vi "D3DM.vi"() -> ()   [LabVIEW 2013]
uses:
  <vilib>/Native 3D Graph/xcontrol/3DPC_SurfacePlot.xctl
  <vilib>/Platform/NI_3dgraph.lvlib
panel:
  out "String":string
  in  "Tab Control":T1(tab)
  in  "mode":enum16{"Manual", "Quad", "Vertical", "Half"}(ring)
  in  "Byte to Read(TCP)":i32=512
  in  "Port":u16=8899
  in  "Log File Path":path=path "E:/Dropbox/StaredProject/Distributed3D/D3DM/raw_log.txt"
  in  "Simulation":bool
  out "Init Status":bool
  in  "User Param 2":i16=3000
  in  "User Param 1":i16=1024
  in  "holder_length":dbl=87.37
  in  "magOffset 1":i16
  in  "magOffset 2":i16=-1725
  in  "Servo":i16[](array[numeric])=[1000, 2000, 600, 2190, 1475]
  in  "ArcStepThreshold":dbl=800000.0
  in  "Least Dis":dbl=240.0
  out "InRange":bool
  out "Points Number":i32
  in  "3D Curve - Lorenz Attractor":refnum<k7>(container)
  in  "Arm Angle Set":i32(slide)=90 min=0 max=180 scale=0.0..180.0
  out "Title":string="      Distributed 3D Measurement Control Panel"
  in  "Initialize":bool
  in  "Base Rotation Speed Set":i32(slide)=1475 min=1000 max=2000 step=1 scale=1000.0..2000.0
  in  "Command":string
  out "Read Buffer":string
  out "help":string="1.Set the target Port number;\n2.Press \"Ready\" button to start acquiring data;\n3.Use arrow keys to control movement;\n4.Use the speed pointer slide to control speed;\n5.Use the Arm Angle slide to control arm;\n6.Press \"ESC\" to stop the car, 3D plot should be     finished automatically.\n\n//quad parameters\nint leftLimit = 1024;\nint rightLimit = 3072;\n//vertical parameters\nint vertical_delay_time = 100;\nint vertical_spd = BASE_STOP + 150;\n//half parameters\nint half_spd = BASE_STOP + 150;\nint half_angle_step = 1;"
  out "3D Graph":refnum<class "Base Datatype.lvclass">[](xcontrol)
  in  "Stop Button":bool
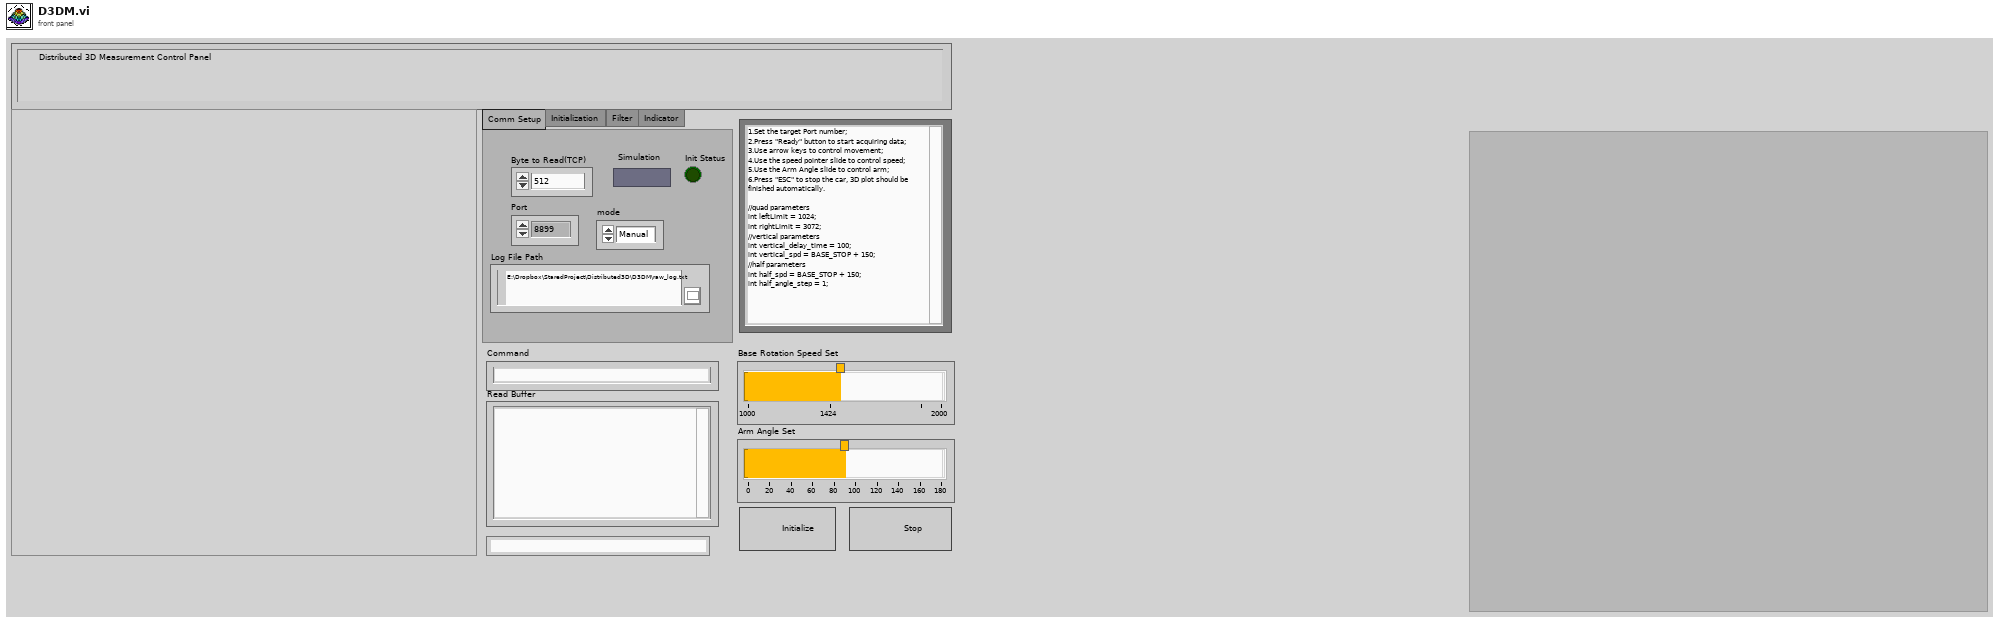
[diagram p1: front panel]
types:
  T1 = enum32{"Comm Setup", "Initialization", "Filter", "Indicator"}
  T2 = enum16{"open", "replace", "create", "open or create", "replace or create", "replace or create with confirmation"}
  T3 = enum16{"Standard", "Buffered", "CRLF", "Immediate"}
  T4 = typedef "eventvkey.ctl" = enum16{"ASCII", "Enter", "Return", "Shift", "Ctrl", "Alt", "Cmd", "Opt", "Caps", "NumLock", "Clear", "Break", "Up", "Down", "Left", "Right", "Insert", "Delete", "Home", "End", "PageUp", "PageDown", "Escape", "Help", "Pause", "ScrollLock", "F1", "F2", "F3", "F4", "F5", "F6", "F7", "F8", "F9", "F10", "F11", "F12", "F13", "F14", "F15", "F16", "F17", "F18", "F19", "F20", "F21", "F22", "F23", "F24", "Play", "VolumeUp", "VolumeDown", "Mute", "Two Byte Char"}
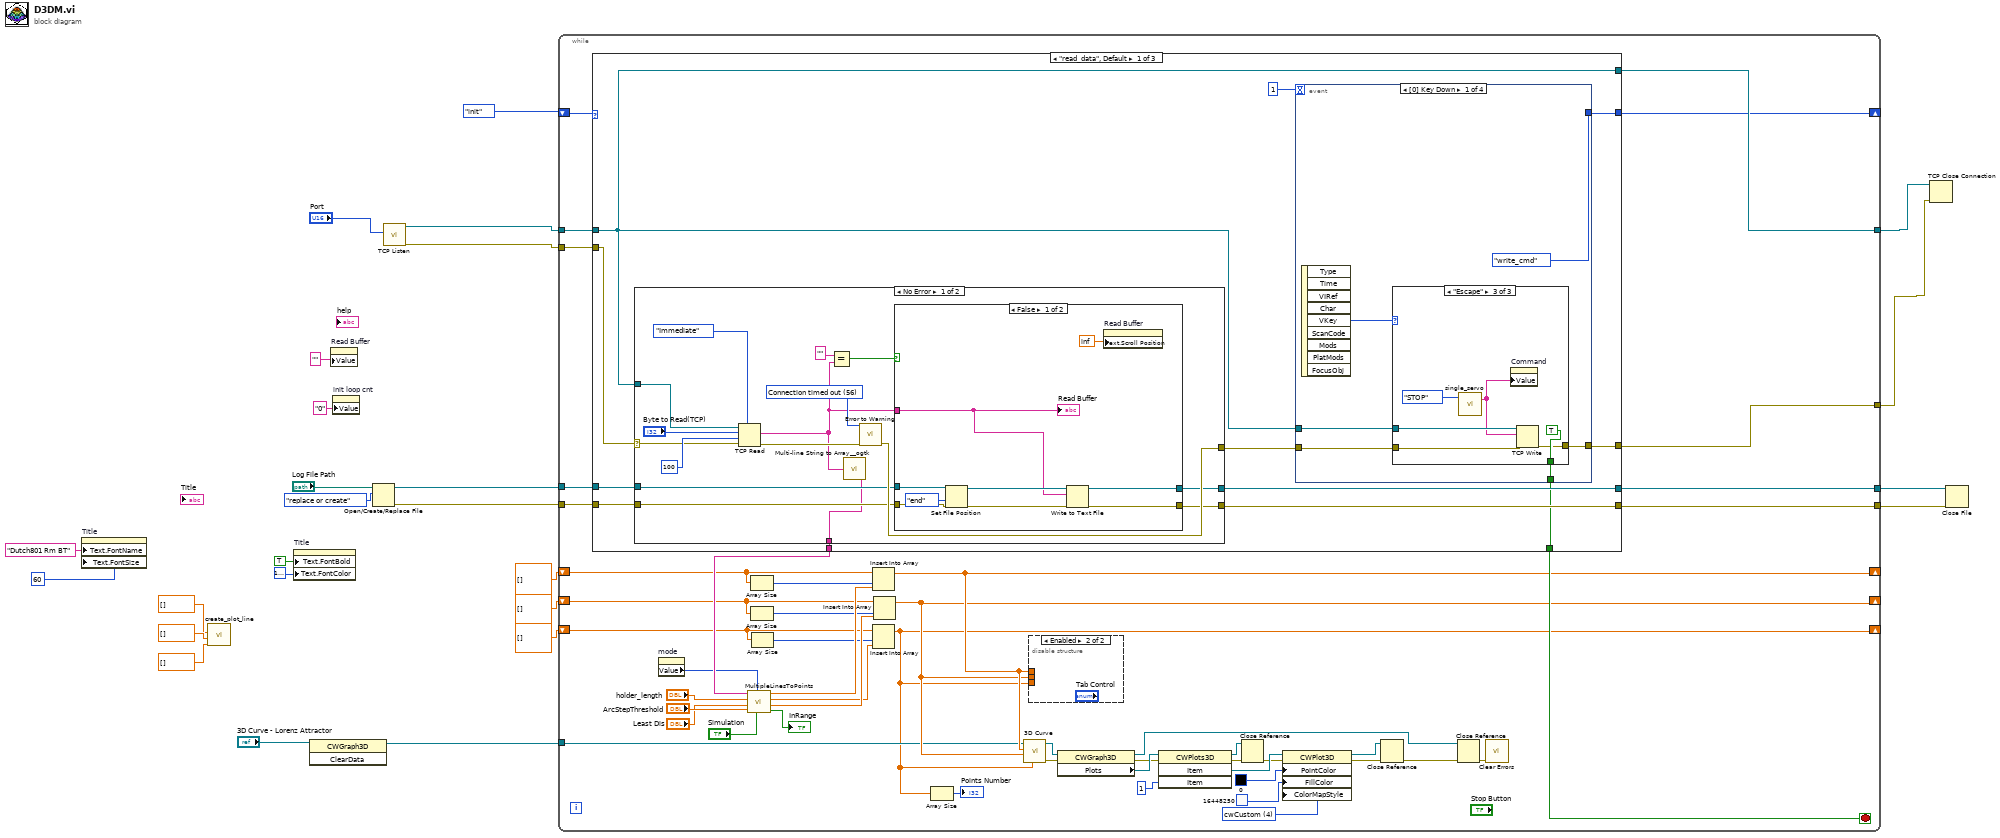
[diagram p0: block diagram]
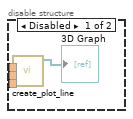
[diagram p2: hidden frame]
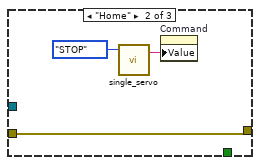
[diagram p4: hidden frame]
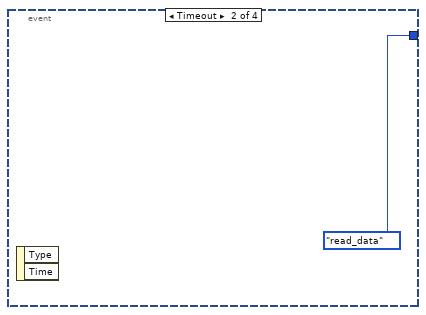
[diagram p5: hidden frame]
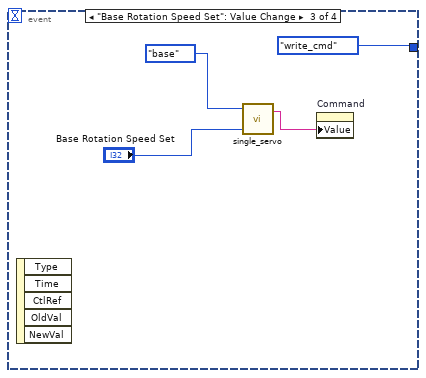
[diagram p6: hidden frame]
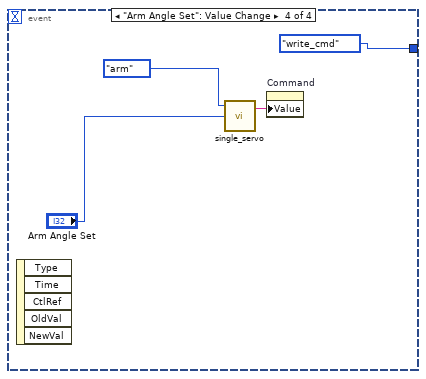
[diagram p7: hidden frame]
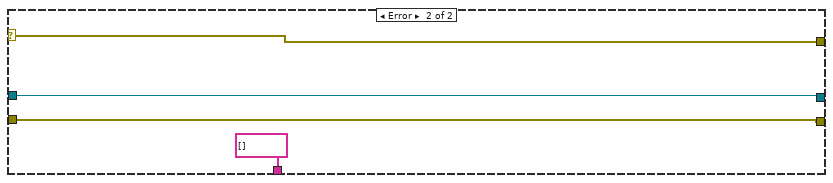
[diagram p9: hidden frame]
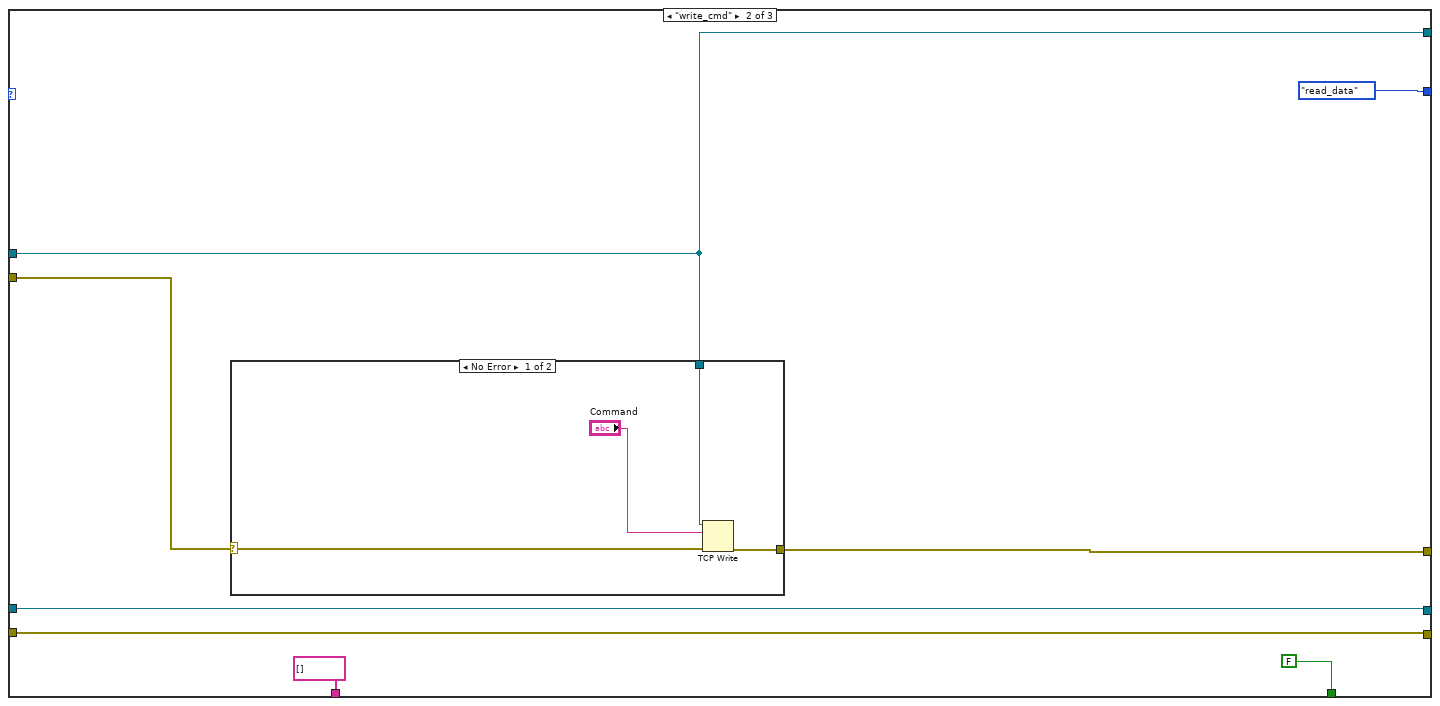
[diagram p10: hidden frame]
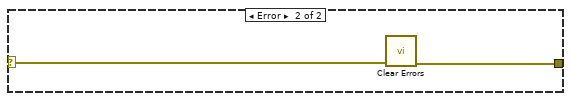
[diagram p11: hidden frame]
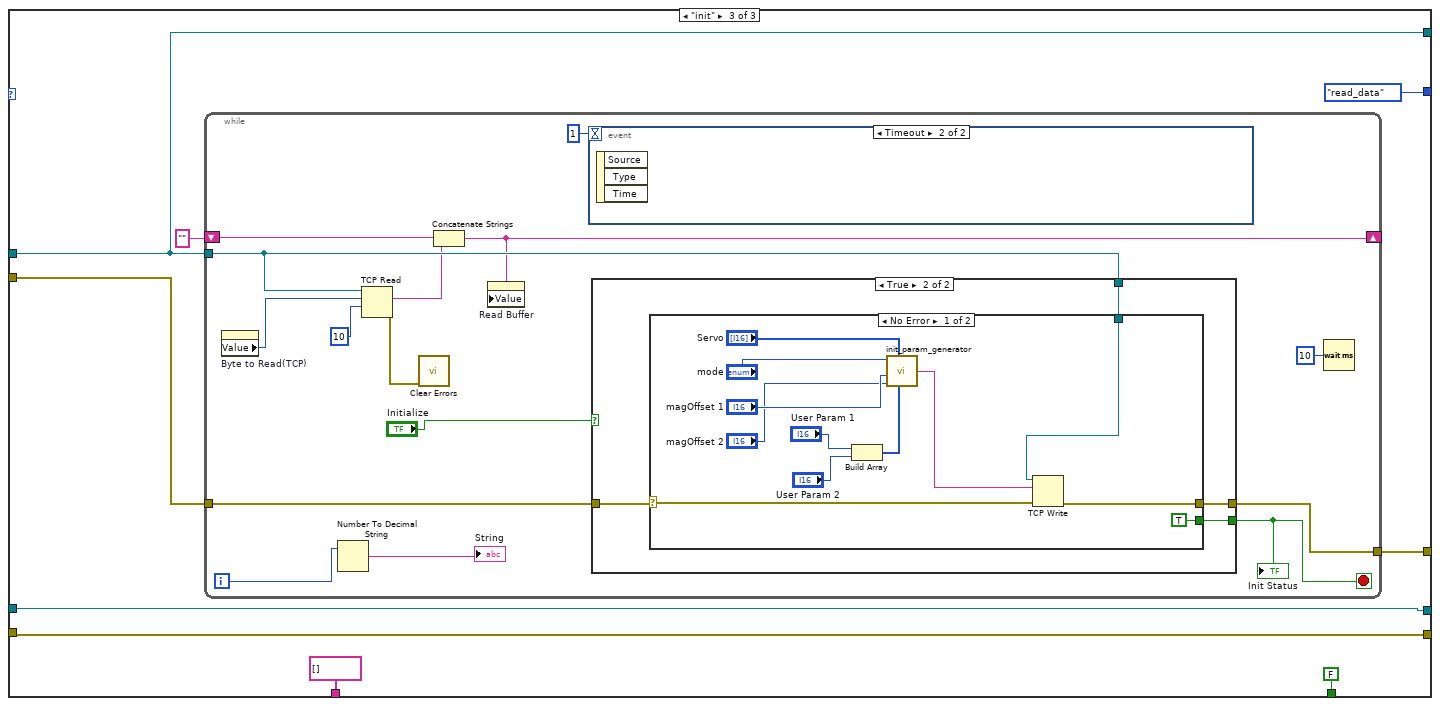
[diagram p12: hidden frame]
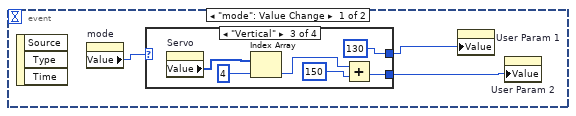
[diagram p13: hidden frame]
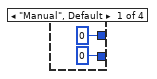
[diagram p14: hidden frame]
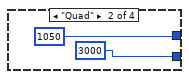
[diagram p15: hidden frame]
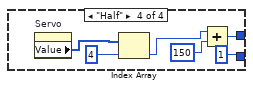
[diagram p16: hidden frame]
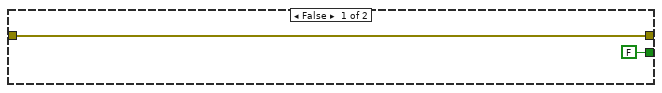
[diagram p17: hidden frame]
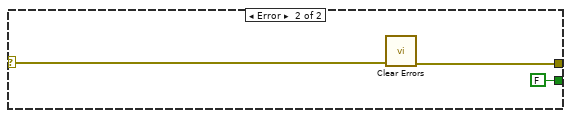
[diagram p18: hidden frame]
diagram:
  n1 = property on="Title" class="Str"("Text.FontName"="Dutch801 Rm BT" ("Text.Font:Name"), "Text.FontSize"=u32 60 ("Text.Font:Size")) -> ()  [unwired: 2 in, 2 out]
  n2 = call <vilib>:"create_plot_line.vi"("z vector"=dbl[] [], "y vector"=dbl[] [], "x vector"=dbl[] []) -> ()  [unwired: 8 in, 1 out]
  n3 = property on="Title" class="Str"("Text.FontBold"=TRUE ("Text.Font:Bold"), "Text.FontColor"=u32 16777222) -> ()  [unwired: 2 in, 2 out]
  n4 = invoke class="CWGraph3D" method="ClearData"(reference="3D Curve - Lorenz Attractor") -> (reference out=w6:refnum<k7>)  [unwired: 2 in, 2 out]
  n5 = property on="Read Buffer" class="Str"("Value"="") -> ()  [unwired: 2 in, 2 out]
  n6 = property on="init loop cnt" class="Str"("Value"="0" ("String")) -> ()  [unwired: 2 in, 2 out]
  n7 = Open/Create/Replace File(file path (use dialog)="Log File Path", operation (0:open)=T2."replace or create") -> (refnum out=w19:refnum<file>, error out=w18:errorcluster)  [unwired: 4 in, 1 out]
  n8 = call <vilib>:"TCP Listen.vi"("port"="Port") -> ("error out"=w24:errorcluster, "connection ID"=w25:refnum<k5>)  [unwired: 6 in, 3 out]
  n9 = while {
    shift-right: [w65] -> _
    shift-left: enum16{"read_data", "write_cmd", "init"}."init" ("RWstate") -> [w75]
    tunnel: w24 -> [w74]
    tunnel: w25 -> [w73]
    tunnel: w19 -> [w72]
    tunnel: w18 -> [w71]
    tunnel: [w70] -> w17
    tunnel: [w69] -> w16
    tunnel: [w67] -> w23
    tunnel: [w66] -> w22
    shift-right: [w39] -> _
    shift-left: dbl[] [] -> [w60]
    shift-right: [w38] -> _
    shift-left: dbl[] [] -> [w56]
    shift-right: [w28] -> _
    shift-left: dbl[] [] -> [w55]
    tunnel: w6 -> [w31]
    stop <- w68 stop-if-true
    w35 = 4 items=["cwNone", "cwShaded", "cwColorSpectrum", "cwGrayScale", "cwCustom"] ("ColorMapStyle")
    n10 = case shown="\"read_data\", Default" w75 {
      tunnel: w74 -> [w91 w155 w170]
      tunnel: w73 -> [w83 w150 w169]
      tunnel: w72 -> [w90 w154 w166]
      tunnel: w71 -> [w89 w153 w165]
      tunnel: [w88 w154 w166] -> w70
      tunnel: [w87 w153 w165] -> w69
      tunnel: [w86 FALSE FALSE] -> w68
      tunnel: [w84 w152 w168] -> w67
      tunnel: [w83 w150 w169] -> w66
      tunnel: [w82 enum16{"read_data", "write_cmd", "init"}."read_data" ("RWstate") enum16{"read_data", "write_cmd", "init"}."read_data" ("RWstate")] -> w65
      tunnel: [w80 string[] [] ("lines") string[] [] ("lines")] -> w61
      frame "read_data", Default {
        n11 = case shown="No Error" w91 {
          selector: w91 -> [w124 w147]
          tunnel: [w128 w147] -> w85
          tunnel: w83 -> [w125 _]
          tunnel: w90 -> [w123 w146]
          tunnel: w89 -> [w122 w145]
          tunnel: [w121 w146] -> w88
          tunnel: [w120 w145] -> w87
          tunnel: [w118 string[] [] ("lines")] -> w80
          frame No Error {
            w132 = 56 items=["No Error", "Argument Error", "Memory Full", "Out of Zone", "End of File", "File Already Open", "Generic File IO Error", "File Not Found", "File Permission Error", "Disk Full", "Duplicate Path", "Too Many Files Open", "Not Enabled", "Resource File Not Found", "Cannot Add Resource", "Resource Not Found", "Image Not Found", "Image Memory Error", "Pen Does Not Exist", "Config Bad Type", "Config Token Not Found", "Config Parse Error", "Config Memory Error", "Bad External Code Format", "Bad External Code Offset", "External Code Not Present", "Null Window", "Destroy Window Mixup", "Null Menu", "Print Aborted", "Bad Print Record", "Print Driver Error", "Windows Error During Print", "Memory Error During Print", "Print Dialog Error", "Generic Print Error", "Invalid Device Refnum", "Device Not Found", "Device Parameter Error", "Device Unit Error", "Can't Open Device", "Device Call Aborted", "Generic Error", "Cancelled By User", "Object ID Too Low", "Object ID Too High", "Object Not In Heap", "Unknown Heap", "Bad DefProc ID", "DefProc Not In Table", "Message Out Of Range", "Null Method", "Unknown Message", "Manager Call Not Supported", "Bad address", "Connection In progress", "Connection timed out", "Connection is already in progress", "Network attribute not supported", "Network error", "Address in use", "System out of memory", "Connection aborted", "Connection refused", "Connection is not connected", "Connection is already connected", "Connection closed", "Initialize error (interapplication manager)", "Bad occurrence", "Wait on unbound occurrence handler", "Occurrence queue overflow", "Bad path", "Semaphore not signaled", "Unrecognized type (interapplication manager)"] ("1st Error to Convert")
            n12 = TCP Read(connection ID=w125, bytes to read="Byte to Read(TCP)", error in (no error)=w124, 7:T3."Immediate" ("mode (standard)"), 9:100) -> (data out=w119:string, error out=w131:errorcluster)  [unwired: 1 out]
            n13 = Equal?(x="", y=w119) -> (x = y?=w127:bool)
            n14 = call <userlib>:"Multi-line String to Array__ogtk.vi"("string"=w119) -> ("lines"=w118:string[])
            n15 = call <vilib>:"Error to Warning.vi"("1st Error to Convert"=w132, "error in"=w131) -> ("warning out"=w128:errorcluster)  [unwired: 13 in]
            n16 = case shown="False" w127 {
              tunnel: w119 -> [w133 _]
              tunnel: w123 -> [w140 w143]
              tunnel: w122 -> [w139 w142]
              tunnel: [w135 w143] -> w121
              tunnel: [w134 w142] -> w120
              frame False {
                n17 = Set File Position(refnum=w140, from (0:start)=enum16{"start", "end", "current"}."end", error in=w139) -> (refnum out=w138:refnum<file>, error out=w137:errorcluster)  [unwired: 1 in]
                n18 = Write to Text File(file (use dialog)=w138, text=w133, error in=w137) -> (refnum out=w135:refnum<file>, error out=w134:errorcluster)  [unwired: 1 in, 1 out]
                n19 = property on="Read Buffer" class="Str"("Text.Scroll Position"=inf) -> ()  [unwired: 2 in, 2 out]
                "Read Buffer" <- w133
              }
              frame True {
              }
            }
          }
          frame Error {
          }
        }
        n20 = event shown="[0] Key Down" {
          selector: _ -> [_ _ _ _]
          dyn-events: _ -> [_ _ _ _]
          timeout: 1 -> [_ _ _ _]
          tunnel: [enum16{"read_data", "write_cmd"}."write_cmd" ("RWstate") enum16{"read_data", "write_cmd"}."read_data" ("RWstate") enum16{"read_data", "write_cmd"}."write_cmd" ("RWstate") enum16{"read_data", "write_cmd"}."write_cmd" ("RWstate")] -> w82
          tunnel: [w96 _ _ _] -> w86
          tunnel: [w94 _ _ _] -> w84
          tunnel: w83 -> [w93 _ _ _]
          tunnel: w85 -> [w92 _ _ _]
          event Key Down {
            n21 = event-data() -> ("VKey"=w95:T4)  [unwired: 1 in, 8 out]
            n22 = case shown="\"Escape\"" w95 {
              tunnel: [_ _ TRUE] -> w96
              tunnel: [w98 w101 w106] -> w94
              tunnel: w93 -> [_ _ w105]
              tunnel: w92 -> [w98 w101 w104]
              frame "ASCII", Default {
              }
              frame "Home" {
                n23 = call "single_servo.vi"("ServoControl"=enum16{"STOP", "both", "arm", "base"}."STOP") -> ("cmd"=w99:string)  [unwired: 3 in]
                n24 = property on="Command" class="Str"("Value"=w99) -> ()  [unwired: 2 in, 2 out]
              }
              frame "Escape" {
                n25 = call "single_servo.vi"("ServoControl"=enum16{"STOP", "both", "arm", "base"}."STOP") -> ("cmd"=w102:string)  [unwired: 3 in]
                n26 = property on="Command" class="Str"("Value"=w102) -> ()  [unwired: 2 in, 2 out]
                n27 = TCP Write(connection ID=w105, data in=w102, error in (no error)=w104) -> (error out=w106:errorcluster)  [unwired: 1 in, 2 out]
              }
            }
          }
          event Timeout {
            n28 = event-data() -> ()  [unwired: 1 in, 2 out]
          }
          event "Base Rotation Speed Set": Value Change {
            n29 = event-data() -> ()  [unwired: 1 in, 5 out]
            n30 = call "single_servo.vi"("base_set"="Base Rotation Speed Set", "ServoControl"=enum16{"STOP", "both", "arm", "base"}."base") -> ("cmd"=w111:string)  [unwired: 2 in]
            n31 = property on="Command" class="Str"("Value"=w111) -> ()  [unwired: 2 in, 2 out]
          }
          event "Arm Angle Set": Value Change {
            n32 = event-data() -> ()  [unwired: 1 in, 5 out]
            n33 = call "single_servo.vi"("arm_set"="Arm Angle Set", "ServoControl"=enum16{"STOP", "both", "arm", "base"}."arm") -> ("cmd"=w115:string)  [unwired: 2 in]
            n34 = property on="Command" class="Str"("Value"=w115) -> ()  [unwired: 2 in, 2 out]
          }
        }
      }
      frame "write_cmd" {
        n35 = case shown="No Error" w155 {
          selector: w155 -> [w158 w160]
          tunnel: [w159 w161] -> w152
          tunnel: w150 -> [w157 _]
          frame No Error {
            n36 = TCP Write(connection ID=w157, data in="Command", error in (no error)=w158) -> (error out=w159:errorcluster)  [unwired: 1 in, 2 out]
          }
          frame Error {
            n37 = call <vilib>:"Clear Errors.vi"("error in (no error)"=w160) -> ("error out"=w161:errorcluster)  [unwired: 6 in]
          }
        }
      }
      frame "init" {
        n38 = while {
          tunnel: w170 -> [w180]
          tunnel: w169 -> [w182]
          tunnel: [w185] -> w168
          shift-right: [w172] -> _
          shift-left: "" -> [w173]
          i -> [w176]
          stop <- w183 stop-if-true
          n39 = property on="Byte to Read(TCP)" class="DigNum (strict)"() -> ("Value"=w181:i32)  [unwired: 2 in, 2 out]
          n40 = Number To Decimal String(number=w176) -> (decimal integer string=→"String":string)  [unwired: 1 in]
          n41 = TCP Read(connection ID=w182, bytes to read=w181, 9:10 ("timeout ms (25000)")) -> (data out=w174:string, error out=w175:errorcluster)  [unwired: 2 in, 1 out]
          n42 = call <vilib>:"Clear Errors.vi"("error in (no error)"=w175) -> ()  [unwired: 6 in, 1 out]
          n43 = Concatenate Strings(w173, w174) -> (w172:string)
          n44 = property on="Read Buffer" class="Str"("Value"=w172) -> ()  [unwired: 2 in, 2 out]
          n45 = event shown="[1] Timeout" {
            selector: _ -> [_ _]
            dyn-events: _ -> [_ _]
            timeout: 1 -> [_ _]
            event "mode": Value Change {
              n46 = event-data() -> ()  [unwired: 1 in, 3 out]
              n47 = property on="mode" class="Enum (strict)"() -> ("Value"=w188:enum16{"Manual", "Quad", "Vertical", "Half"})  [unwired: 2 in, 2 out]
              n48 = case shown="\"Vertical\"" w188 {
                tunnel: [i16 0 i16 1050 i16 130 w200] -> w187
                tunnel: [i16 0 i16 3000 w193 i16 1] -> w186
                frame "Manual", Default {
                }
                frame "Quad" {
                }
                frame "Vertical" {
                  n49 = property on="Servo" class="Arr (strict)"() -> ("Value"=w198:i16[])  [unwired: 2 in, 2 out]
                  n50 = Index Array(array=w198, index=4) -> (element=w195:i16)
                  n51 = Add(x=w195, y=i16 150) -> (x+y=w193:i16)
                }
                frame "Half" {
                  n52 = property on="Servo" class="Arr (strict)"() -> ("Value"=w204:i16[])  [unwired: 2 in, 2 out]
                  n53 = Index Array(array=w204, index=4) -> (element=w201:i16)
                  n54 = Add(x=w201, y=i16 150) -> (x+y=w200:i16)
                }
              }
              n55 = property on="User Param 1" class="DigNum (strict)"("Value"=w187) -> ()  [unwired: 2 in, 2 out]
              n56 = property on="User Param 2" class="DigNum (strict)"("Value"=w186) -> ()  [unwired: 2 in, 2 out]
            }
            event Timeout {
              n57 = event-data() -> ()  [unwired: 1 in, 3 out]
            }
          }
          n58 = case shown="True" "Initialize" {
            tunnel: [w206 w210] -> w185
            tunnel: [FALSE ("status") w209] -> w183
            tunnel: w182 -> [_ w208]
            tunnel: w180 -> [w206 w207]
            frame False {
            }
            frame True {
              n59 = case shown="No Error" w207 {
                selector: w207 -> [w222 w224]
                tunnel: [w219 w225] -> w210
                tunnel: w208 -> [w221 _]
                tunnel: [TRUE ("status") FALSE ("status")] -> w209
                frame No Error {
                  n60 = Build Array("User Param 1", "User Param 2") -> (w213:i16[])
                  n61 = call "init_param_generator.vi"("Limit"=w213, "Servo"="Servo", "mag offset 2"="magOffset 2", "mag offset 1"="magOffset 1", "mode"="mode") -> ("init param"=w220:string)  [unwired: 1 in]
                  n62 = TCP Write(connection ID=w221, data in=w220, error in (no error)=w222) -> (error out=w219:errorcluster)  [unwired: 1 in, 2 out]
                }
                frame Error {
                  n63 = call <vilib>:"Clear Errors.vi"("error in (no error)"=w224) -> ("error out"=w225:errorcluster)  [unwired: 6 in]
                }
              }
            }
          }
          "Init Status" <- w183
          n64 = Wait (ms)(milliseconds to wait=u32 10) -> ()  [unwired: 1 out]
        }
      }
    }
    n65 = property on="mode" class="Enum (strict)"() -> ("Value"=w29:enum16{"Manual", "Quad", "Vertical", "Half"})  [unwired: 2 in, 2 out]
    n66 = call "MultipleLinesToPoints.vi"("Sim"="Simulation", "mode"=w29, "Arc Threshold"="ArcStepThreshold", "Least Dis"="Least Dis", "holder_length"="holder_length", "lines"=w61) -> ("InRange"=→"InRange":bool, "y"=w63:dbl[], "z"=w62:dbl[], "x"=w64:dbl[])
    n67 = Array Size(array=w60) -> (size(s)=w59:i32)
    n68 = Array Size(array=w56) -> (size(s)=w58:i32)
    n69 = Array Size(array=w55) -> (size(s)=w57:i32)
    n70 = Insert Into Array(array=w60, index=w59, new element=w64) -> (w39:dbl[])
    n71 = Insert Into Array(array=w55, index=w57, new element=w62) -> (w28:dbl[])
    n72 = Insert Into Array(array=w56, index=w58, new element=w63) -> (w38:dbl[])
    n73 = Array Size(array=w28) -> (size(s)=→"Points Number":i32)
    n74 = call <vilib>:"3D Curve.vi"("z vector"=w28, "y vector"=w38, "x vector"=w39, "3D graph"=w31) -> ("error out"=w51:errorcluster, "3D graph out"=w50:refnum<k7>)  [unwired: 6 in]
    n75 = disable-structure shown="Enabled" {
      disable-tunnel: w39 -> [w78 _]
      disable-tunnel: w38 -> [w77 _]
      disable-tunnel: w28 -> [w76 _]
      frame Disabled {
        n76 = call <vilib>:"create_plot_line.vi"("z vector"=w76, "y vector"=w77, "x vector"=w78) -> ("plots out"=→"3D Graph":refnum<class "Base Datatype.lvclass">[])  [unwired: 8 in]
      }
      frame Enabled {
      }
    }
    n77 = property class="CWGraph3D"(reference=w50, error in=w51) -> (reference out=w41:refnum<k7>, error out=w49:errorcluster, "Plots"=w53:refnum<k7>)
    n78 = invoke class="CWPlots3D" method="Item"(reference=w53, error in=w49, "Item"=1) -> (reference out=w47:refnum<k7>, error out=w48:errorcluster, "Item"=w52:refnum<k7>)  [unwired: 1 in, 1 out]
    n79 = Close Reference(reference=w47, error in (no error)=w48) -> (error out=w46:errorcluster)
    n80 = property class="CWPlot3D"(reference=w52, error in=w46, "PointColor"=u32 0, "FillColor"=u32 16448250, "ColorMapStyle"=w35) -> (reference out=w44:refnum<k7>, error out=w45:errorcluster)
    n81 = Close Reference(reference=w44, error in (no error)=w45) -> (error out=w42:errorcluster)
    n82 = Close Reference(reference=w41, error in (no error)=w42) -> (error out=w43:errorcluster)
    n83 = call <vilib>:"Clear Errors.vi"("error in (no error)"=w43) -> ()  [unwired: 6 in, 1 out]
  }
  n84 = TCP Close Connection(connection ID=w22, error in (no error)=w23) -> ()  [unwired: 1 in, 2 out]
  n85 = Close File(refnum=w17, error in=w16) -> ()  [unwired: 2 out]
